vi "ValueSignalByPathArray.vi"(0 "VI Reference In":refnum<vi>, 5 "Control Path":string[](array[string]), 7 "Value (Signaling)":variant, 11 "error in":errorcluster) -> (4 "VI Reference Out":refnum<vi>, 6 "Ctl Reference Out":refnum<vi>, 15 "error out":errorcluster)   [LabVIEW 2016, in "Drona.lvlib" / "ControlValue.lvlib"]
doc: "Sets the value of control which is specified.\n\nThe path of the control should be given in the successive index of the array"
uses:
  ControlValue.lvlib
  Get/GetControlRef/GetControlRef.lvlib
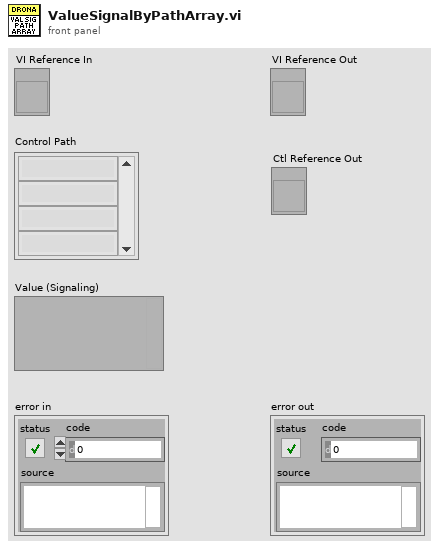
[diagram p1: front panel]
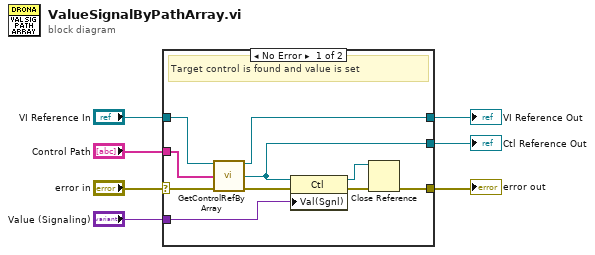
[diagram p0: block diagram]
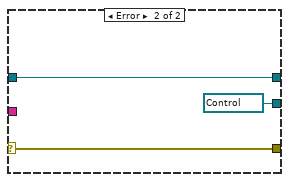
[diagram p2: hidden frame]
diagram:
  n1 = case shown="No Error" "error in" {
    selector: "error in" -> [w16 w20]
    tunnel: "Control Path" -> [w13 _]
    tunnel: "VI Reference In" -> [w12 w19]
    tunnel: [w9 w19] -> w4
    tunnel: "Value (Signaling)" -> [w17 _]
    tunnel: [w11 w20] -> w2
    tunnel: [w8 refnum<vi> refnum ("Ctl Refnum")] -> w1
    frame No Error {
      # "Target control is found and value is set"
      n2 = call "GetControlRefByArray.vi"("VI Reference In"=w12, "Control Path"=w13, "error In"=w16) -> ("VI Reference Out"=w9:refnum<vi>, "Ctl Refnum"=w8:refnum<vi>, "error out"=w15:errorcluster)  [unwired: 10 in]
      n3 = property class="Ctl"(reference=w8, error in=w15, "Val(Sgnl)"=w17) -> (reference out=w10:refnum<vi>, error out=w14:errorcluster)
      n4 = Close Reference(reference=w10, error in (no error)=w14) -> (error out=w11:errorcluster)
    }
    frame Error {
    }
  }
  "error out" <- w2
  "VI Reference Out" <- w4
  "Ctl Reference Out" <- w1
